vi "Write data for storage.vi"(7 "Application path":path, 8 "Error In":errorcluster, 9 "Humidity":dbl, 10 "Temperature":dbl, 11 "MAC address":string) -> (0 "Error Out":errorcluster, 2 "Result":string)   [LabVIEW 2016]
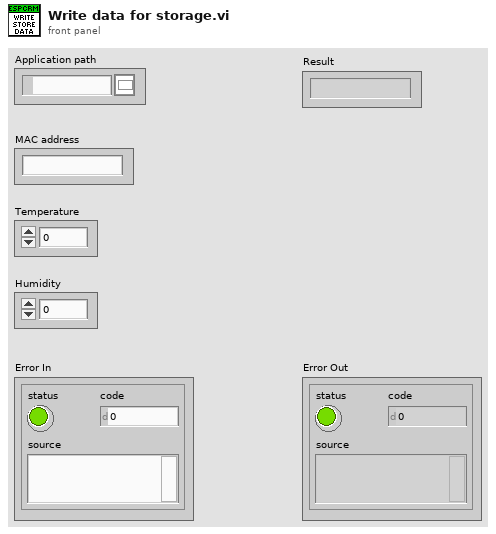
[diagram p1: front panel]
types:
  T1 = enum16{"open", "replace", "create", "open or create", "replace or create", "replace or create with confirmation"}
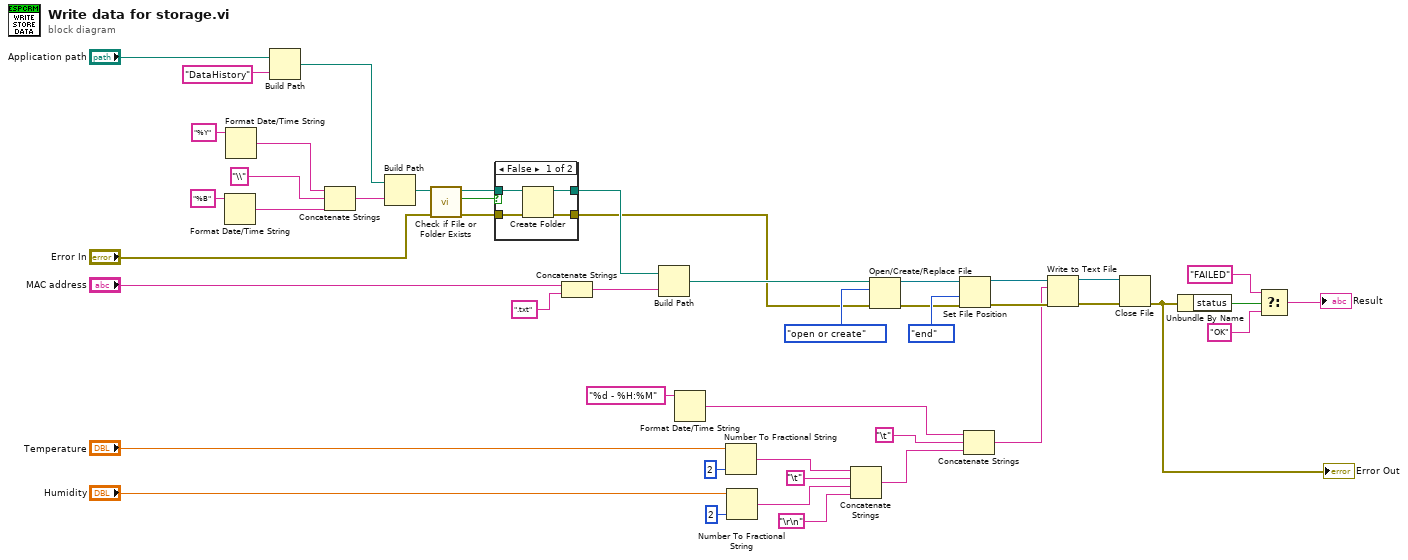
[diagram p0: block diagram]
diagram:
  n1 = Format Date/Time String(time format string (%c)="%B") -> (date/time string=w29:string)  [unwired: 2 in]
  n2 = Format Date/Time String(time format string (%c)="%Y") -> (date/time string=w31:string)  [unwired: 2 in]
  n3 = Build Path(base path="Application path", name or relative path="DataHistory") -> (appended path=w20:path)
  n4 = Concatenate Strings(w31, "\\" ("string"), w29) -> (w34:string)
  n5 = Build Path(base path=w20, name or relative path=w34) -> (appended path=w28:path)
  n6 = call <vilib>:"Check if File or Folder Exists.vi"("error in (no error)"="Error In", "path"=w28) -> ("error out"=w27:errorcluster, "file or folder exists?"=w25:bool, "dup path"=w26:path)  [unwired: 7 in]
  n7 = case shown="False" w25 {
    tunnel: w27 -> [w50 w51]
    tunnel: w26 -> [w49 w52]
    tunnel: [w48 w52] -> w24
    tunnel: [w47 w51] -> w17
    frame False {
      n8 = Create Folder(path (use dialog)=w49, error in=w50) -> (created path=w48:path, error out=w47:errorcluster)  [unwired: 1 in, 1 out]
    }
    frame True {
    }
  }
  n9 = Concatenate Strings("MAC address", ".txt" ("string")) -> (w22:string)
  n10 = Build Path(base path=w24, name or relative path=w22) -> (appended path=w21:path)
  n11 = Format Date/Time String(time format string (%c)="%d - %H:%M") -> (date/time string=w10:string)  [unwired: 2 in]
  n12 = Number To Fractional String(number="Temperature", precision (6)=i16 2) -> (F-format string=w16:string)  [unwired: 2 in]
  n13 = Number To Fractional String(number="Humidity", precision (6)=i16 2) -> (F-format string=w15:string)  [unwired: 2 in]
  n14 = Concatenate Strings(w16, "\t", w15, "\r\n") -> (w9:string)
  n15 = Open/Create/Replace File(file path (use dialog)=w21, error in=w17, operation (0:open)=T1."open or create") -> (refnum out=w39:refnum<file>, error out=w37:errorcluster)  [unwired: 3 in, 1 out]
  n16 = Set File Position(refnum=w39, from (0:start)=enum16{"start", "end", "current"}."end", error in=w37) -> (refnum out=w35:refnum<file>, error out=w36:errorcluster)  [unwired: 1 in]
  n17 = Concatenate Strings(w10, "\t", w9) -> (w6:string)
  n18 = Write to Text File(file (use dialog)=w35, text=w6, error in=w36) -> (refnum out=w46:refnum<file>, error out=w45:errorcluster)  [unwired: 1 in, 1 out]
  n19 = Close File(refnum=w46, error in=w45) -> (error out=w3:errorcluster)  [unwired: 1 out]
  "Error Out" <- w3
  n20 = Unbundle By Name(w3) -> ("status"=w43:bool)
  n21 = Select(t="FAILED", s=w43, f="OK") -> (s? t:f=→"Result":string)
